vi "myRIO__TCP_constants_byteRange_messageType_analogInput.vi"() -> (2 "output_analogInput_byte":u8=73, 3 "output_analogInput_char":string="I")   [LabVIEW 2014]
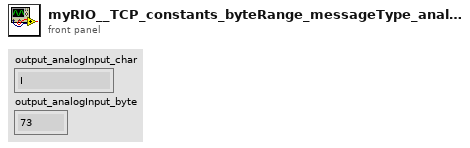
[diagram p1: front panel]
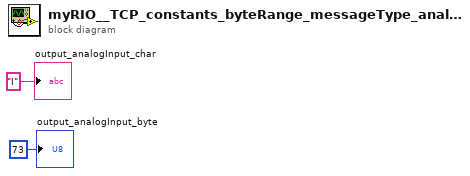
[diagram p0: block diagram]
diagram:
  "output_analogInput_char" <- "I"
  "output_analogInput_byte" <- u8 73
